vi "StayAtHeight.vi"(7 "Description":string, 8 "Command Info In":T1, 9 "Setpoint":dbl) -> (0 "Command Info Out":T1)   [LabVIEW 2018]
doc: "This template includes code for deadband comparision to avoid excessive command scheduling. It is particularly useful for joystick-driven commands.\n\nBe sure to right-click and select New from Template and save with a new command name."
uses:
  <vilib>/Rock Robotics/WPI/Framework/Command Status Info.ctl
  <vilib>/Rock Robotics/WPI/Framework/Completion Status.ctl
  <vilib>/Rock Robotics/WPI/Framework/Completion Notifier.ctl
  Implementation/Elevator Operations.ctl
  Implementation/Elevator Setpoints.ctl
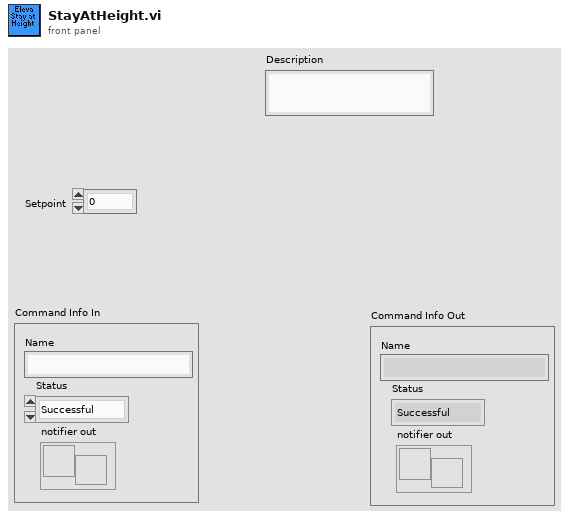
[diagram p1: front panel]
types:
  T1 = typedef "Command Status Info.ctl" = cluster{"Name":string, "Status":T2, "notifier out":T3}
  T2 = typedef "Completion Status.ctl" = enum16{"Successful", "Aborted", "Incomplete"}
  T3 = typedef "Completion Notifier.ctl" = refnum<notifier>
  T4 = typedef "Elevator Operations.ctl" = enum16{"Reserve", "Read Current", "Immediate", "GoToHeight", "StayAtHeight", "LiftForTime"}
  T5 = typedef "Elevator Setpoints.ctl" = cluster{"Operation":T4, "Setpoint":dbl, "Duration":dbl, "Button":bool}
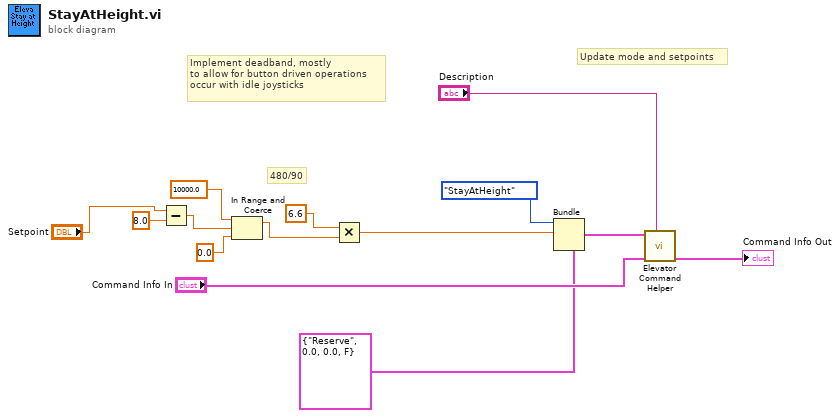
[diagram p0: block diagram]
diagram:
  # "480/90"
  # "Implement deadband, mostly\nto allow for button driven operations\noccur with idle joysticks"
  # "Update mode and setpoints"
  n1 = Subtract(x="Setpoint", y=8.0) -> (x-y=w5:dbl)
  n2 = In Range and Coerce(upper limit=10000.0, x=w5, lower limit=0.0) -> (coerced(x)=w1:dbl)  [unwired: 1 out]
  n3 = Multiply(x=6.6, y=w1) -> (x*y=w7:dbl)
  n4 = Bundle(cluster=T5 {"Operation"=enum."Reserve", "Setpoint"=0.0, "Duration"=0.0, "Button"=FALSE} ("SubSystem Data"), "Operation"=Elevator_Operations."StayAtHeight", "Setpoint"=w7) -> (w10:T5)  [unwired: 2 in]
  n5 = call "Elevator Command Helper.vi"("Description"="Description", "Command Info In"="Command Info In", "SubSystem Data"=w10) -> ("Command Info Out"=→"Command Info Out":T1)  [unwired: 6 in, 2 out]
